vi "ConfigDialog.vi"(8 "error in (no error)":errorcluster, 11 "SamplerPluginsBase in":refnum<class "SamplerPluginsBase.lvclass">) -> (0 "error out":errorcluster, 3 "SamplerPluginsBase out":refnum<class "SamplerPluginsBase.lvclass">)   [LabVIEW 2014, in "SamplerPlugins.lvlib" / "SamplerPluginsBase.lvclass"]
uses:
  SamplerPluginsBase.lvclass
panel:
  in  "Trigger Edge":u16(ring)=10280 items=["Rising"=10280, "Falling"=10171]
  in  "Trigger Source":string
  in  "iSampleCount":i32 caption="Sample Count"
  in  "btnCancel":bool
  in  "btnDone":bool
  in  "eTriggerSource":u16(ring)=1 caption="Trigger Type" items=["NULL", "Immediate", "External", "Software Trigger"]
  in  "iTriggerCount":i32 caption="Trigger Count"
  in  "dSampleRate":dbl caption="Sample Rate"
  in  "eSampleClock":u16(ring) caption="Sample Clock" items=["NULL"=0, "Immediate"=1, "External"=2, "Software Trigger"=3, "Interval"=10]
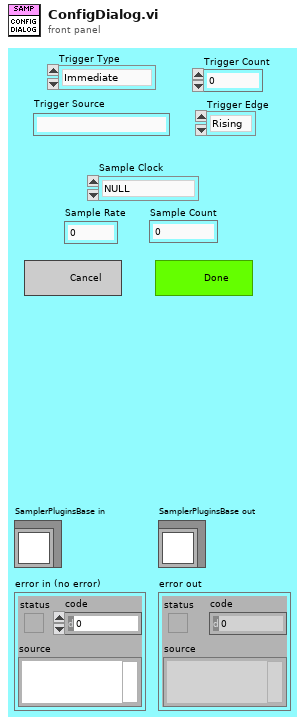
[diagram p1: front panel]
types:
  T1 = enum32{"Invalid", "Default", "Floating", "Floating/Auto-Hide", "Modal"}
  T2 = typedef "SamplerPlugins.lvlib/SamplerPluginsBase.lvclass/ConfigMultiPointParams.ctl" = cluster{"iTriggerCount":i32, "iSampleCount":i32, "eSampleClock":u16, "dSampleInterval":dbl}
  T3 = typedef "SamplerPlugins.lvlib/SamplerPluginsBase.lvclass/MultiPointParams.ctl" = cluster{"iMaxTimeMilliseconds":i32, "iArraySize":i32}
  T4 = typedef "SamplerPlugins.lvlib/SamplerPluginsBase.lvclass/TriggerParams.ctl" = cluster{"eEdge":u16, "sSource":string}
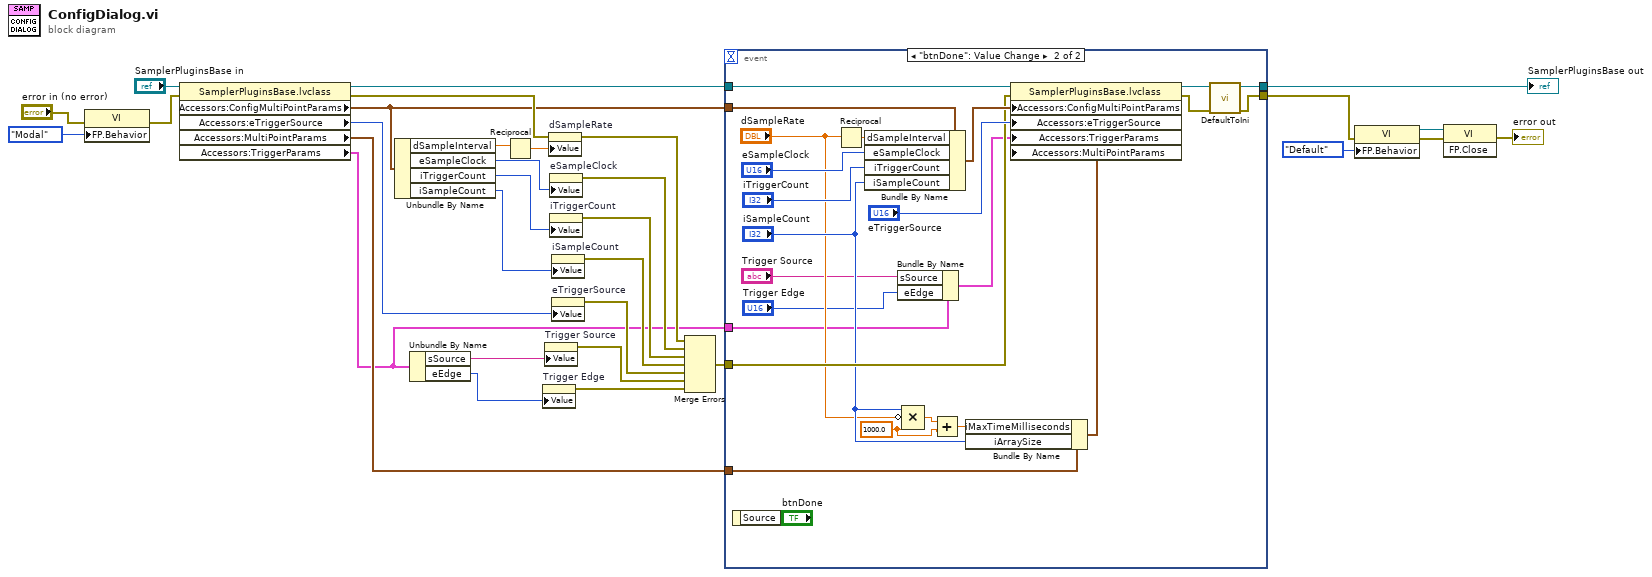
[diagram p0: block diagram]
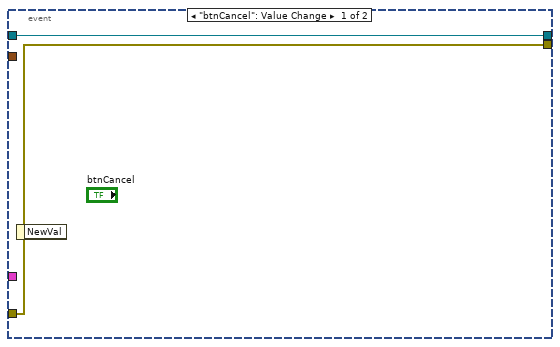
[diagram p2: hidden frame]
diagram:
  n1 = property class="VI"(error in="error in (no error)", "FP.Behavior"=T1."Modal" ("Front Panel Window:Behavior")) -> (error out=w22:errorcluster)  [unwired: 1 in, 1 out]
  n2 = property class="SamplerPluginsBase.lvclass"(reference="SamplerPluginsBase in", error in=w22) -> (reference out=w14:refnum<class "SamplerPluginsBase.lvclass">, error out=w28:errorcluster, "Accessors:ConfigMultiPointParams"=w13:T2, "Accessors:eTriggerSource"=w25:u16, "Accessors:MultiPointParams"=w6:T3, "Accessors:TriggerParams"=w1:T4)
  n3 = Unbundle By Name(w13) -> ("dSampleInterval"=w30:dbl, "eSampleClock"=w27:u16, "iTriggerCount"=w26:i32, "iSampleCount"=w7:i32)
  n4 = Unbundle By Name(w1) -> ("sSource"=w5:string, "eEdge"=w4:u16)
  n5 = Reciprocal(x=w30) -> (1/x=w29:dbl)
  n6 = property on="Trigger Edge" class="Ring (strict)"("Value"=w4) -> (error out=w2:errorcluster)  [unwired: 2 in, 1 out]
  n7 = property on="Trigger Source" class="Str"("Value"=w5) -> (error out=w3:errorcluster)  [unwired: 2 in, 1 out]
  n8 = property on="dSampleRate" class="DigNum (strict)"(error in=w28, "Value"=w29) -> (error out=w19:errorcluster)  [unwired: 1 in, 1 out]
  n9 = property on="eSampleClock" class="Ring (strict)"("Value"=w27) -> (error out=w20:errorcluster)  [unwired: 2 in, 1 out]
  n10 = property on="iTriggerCount" class="DigNum (strict)"("Value"=w26) -> (error out=w21:errorcluster)  [unwired: 2 in, 1 out]
  n11 = property on="iSampleCount" class="DigNum (strict)"("Value"=w7) -> (error out=w8:errorcluster)  [unwired: 2 in, 1 out]
  n12 = property on="eTriggerSource" class="Ring (strict)"("Value"=w25) -> (error out=w9:errorcluster)  [unwired: 2 in, 1 out]
  n13 = Merge Errors(w19, w20, w21, w8, w9, w3, w2) -> (w12:errorcluster)
  n14 = event shown="[1] \"btnDone\": Value Change" {
    selector: _ -> [_ _]
    dyn-events: _ -> [_ _]
    timeout: _ -> [_ _]
    tunnel: w14 -> [w33 w52]
    tunnel: w13 -> [_ w56]
    tunnel: w12 -> [w32 w49]
    tunnel: [w33 w46] -> w11
    tunnel: [w32 w45] -> w10
    tunnel: w6 -> [_ w44]
    tunnel: w1 -> [_ w38]
    event "btnCancel": Value Change {
      n15 = event-data() -> ()  [unwired: 1 in, 1 out]
    }
    event "btnDone": Value Change {
      w39 = 1000.0 ("value")
      n16 = event-data() -> ()  [unwired: 1 in, 1 out]
      n17 = Reciprocal(x="dSampleRate") -> (1/x=w55:dbl)
      n18 = Bundle By Name(cluster=w56, "dSampleInterval"=w55, "eSampleClock"="eSampleClock", "iTriggerCount"="iTriggerCount", "iSampleCount"="iSampleCount") -> (w51:T2)
      n19 = Bundle By Name(cluster=w38, "sSource"="Trigger Source", "eEdge"="Trigger Edge") -> (w34:T4)
      n20 = Compound Arithmetic op=MULTIPLY("iSampleCount", invert "dSampleRate", w39) -> (w41:dbl)
      n21 = Add(x=w41, y=w39) -> (x+y=w40:dbl)
      n22 = Bundle By Name(cluster=w44, "iMaxTimeMilliseconds"=w40, "iArraySize"="iSampleCount") -> (w35:T3)
      n23 = property class="SamplerPluginsBase.lvclass"(reference=w52, error in=w49, "Accessors:ConfigMultiPointParams"=w51, "Accessors:eTriggerSource"="eTriggerSource", "Accessors:TriggerParams"=w34, "Accessors:MultiPointParams"=w35) -> (reference out=w48:refnum<class "SamplerPluginsBase.lvclass">, error out=w47:errorcluster)
      n24 = call-dynamic "DefaultToIni.vi"("error in (no error)"=w47, "SamplerPluginsBase in"=w48) -> ("error out"=w45:errorcluster, "SamplerPluginsBase out"=w46:refnum<class "SamplerPluginsBase.lvclass">)  [unwired: 8 in]
    }
  }
  "SamplerPluginsBase out" <- w11
  n25 = property class="VI"(error in=w10, "FP.Behavior"=T1."Default" ("Front Panel Window:Behavior")) -> (reference out=w18:refnum<vi>, error out=w17:errorcluster)  [unwired: 1 in]
  n26 = invoke class="VI" method="FP.Close"(reference=w18, error in=w17) -> (error out=→"error out":errorcluster)  [unwired: 1 in, 2 out]
